vi "Set Arm.vi"(5 "Override Angle":dbl, 7 "Override Control":T1(ring), 10 "Manual Arm Angle":dbl, 11 "Arm Mode":T2=enum."Disabled") -> ()   [LabVIEW 2015]
uses:
  Arm Mode TypeDef.ctl
  Arm Notifier TypeDef.ctl
  Global Variables.vi
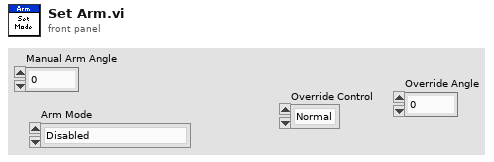
[diagram p1: front panel]
types:
  T1 = enum16{"Normal", "Make arm greater than override angle", "Make arm less than override angle"}
  T2 = typedef "Arm Mode TypeDef.ctl" = enum16{"Unknown", "Disabled", "Locked", "Shoot Batter", "Shoot Close", "Cross Defense", "Human Player Load", "Low Bar / Goal", "Manual"}
  T3 = typedef "Arm Notifier TypeDef.ctl" = cluster{"Arm Mode":T2, "Manual Arm Angle":dbl}
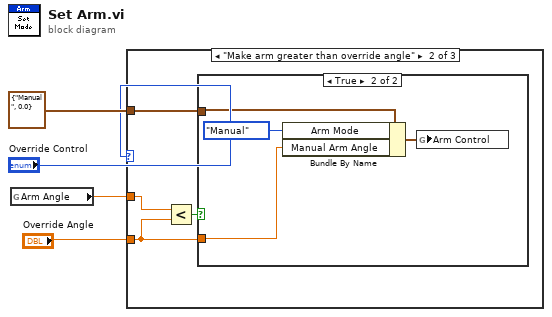
[diagram p0: block diagram]
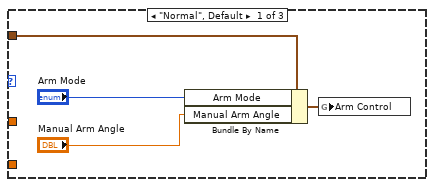
[diagram p2: hidden frame]
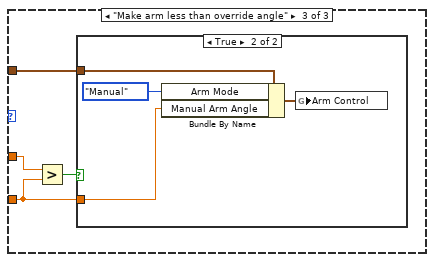
[diagram p4: hidden frame]
diagram:
  n1 = global read "Global Variables.vi" "Arm Angle"() -> (w2:dbl)
  n2 = case shown="\"Make arm greater than override angle\"" "Override Control" {
    tunnel: T3 {"Arm Mode"=enum."Manual", "Manual Arm Angle"=0.0} ("Arm Control") -> [w8 w10 w20]
    tunnel: w2 -> [_ w12 w18]
    tunnel: "Override Angle" -> [_ w9 w17]
    frame "Normal", Default {
      n3 = Bundle By Name(cluster=w8, "Arm Mode"="Arm Mode", "Manual Arm Angle"="Manual Arm Angle") -> (w7:T3)
      n4 = global write "Global Variables.vi" "Arm Control"(w7) -> ()
    }
    frame "Make arm greater than override angle" {
      n5 = Less?(x=w12, y=w9) -> (x < y?=w11:bool)
      n6 = case shown="True" w11 {
        tunnel: w10 -> [_ w15]
        tunnel: w9 -> [_ w13]
        frame False {
        }
        frame True {
          n7 = Bundle By Name(cluster=w15, "Arm Mode"=Arm_Mode_TypeDef."Manual", "Manual Arm Angle"=w13) -> (w16:T3)
          n8 = global write "Global Variables.vi" "Arm Control"(w16) -> ()
        }
      }
    }
    frame "Make arm less than override angle" {
      n9 = Greater?(x=w18, y=w17) -> (0:w19:bool)
      n10 = case shown="True" w19 {
        tunnel: w20 -> [_ w23]
        tunnel: w17 -> [_ w21]
        frame False {
        }
        frame True {
          n11 = Bundle By Name(cluster=w23, "Arm Mode"=Arm_Mode_TypeDef."Manual", "Manual Arm Angle"=w21) -> (w24:T3)
          n12 = global write "Global Variables.vi" "Arm Control"(w24) -> ()
        }
      }
    }
  }
